vi "HEWH Reset Flow Meter.vi"(6 "Refnum in":T1, 7 "Use Emerson 5700":bool, 8 "error in (no error)":errorcluster, 9 "Debug":bool, 10 "Laurel Hot IP Address":string, 11 "dup VISA session in":refnum<visa-resource-name>) -> (0 "error out":errorcluster, 3 "VISA Refnum out":refnum<visa-resource-name>)   [LabVIEW 2016]
uses:
  Drivers/Laurel Meter/Type Definitions/Laurel Serial Commands.ctl
  Drivers/Emerson 5700 Transmitter/Type Definitions/Emerson 5700 Modbus Write Coils.ctl
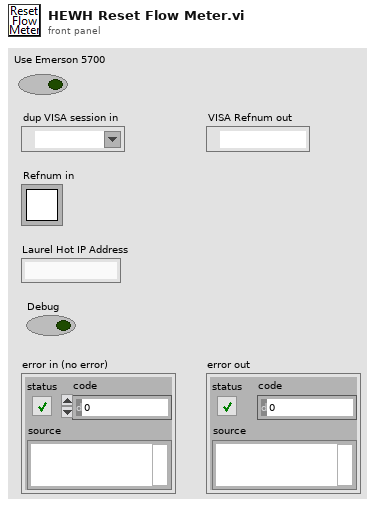
[diagram p1: front panel]
types:
  T1 = typedef "Semaphore RefNum" = refnum<k1>
  T2 = typedef "Laurel Serial Commands.ctl" = string
  T3 = enum16{"Computation Start", "Computation stop", "Reset Computation", "Clear Computation"}
  T4 = typedef "Emerson 5700 Modbus Write Coils.ctl" = u16
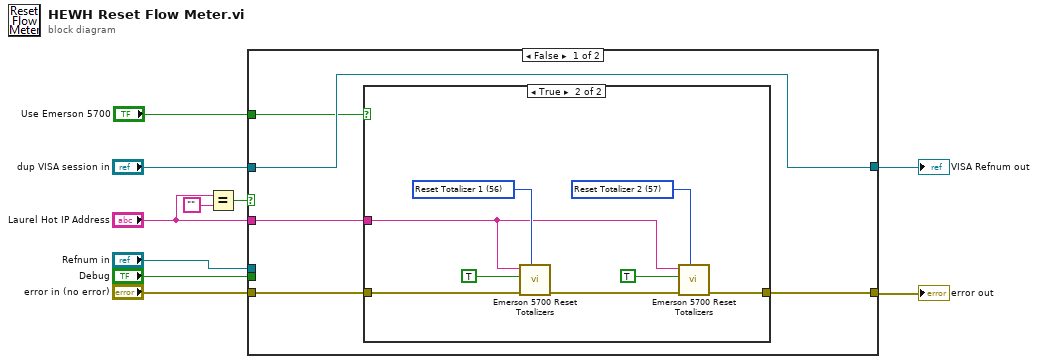
[diagram p0: block diagram]
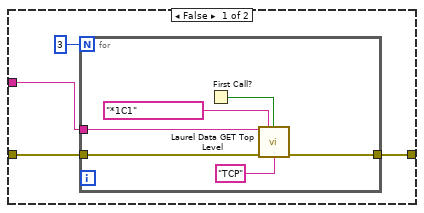
[diagram p2: hidden frame]
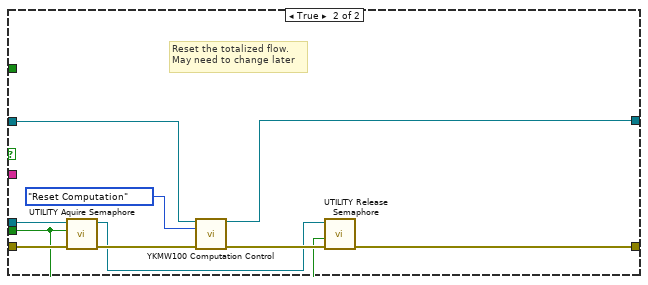
[diagram p3: hidden frame]
diagram:
  n1 = Equal?(x="Laurel Hot IP Address", y="") -> (x = y?=w3:bool)
  n2 = case shown="False" w3 {
    tunnel: "Laurel Hot IP Address" -> [w15 _]
    tunnel: "error in (no error)" -> [w14 w39]
    tunnel: [w13 w38] -> w6
    tunnel: "dup VISA session in" -> [w12 w37]
    tunnel: [w12 w36] -> w8
    tunnel: "Refnum in" -> [_ w35]
    tunnel: "Debug" -> [_ w34]
    tunnel: "Use Emerson 5700" -> [w11 _]
    frame False {
      n3 = case shown="True" w11 {
        tunnel: w15 -> [w18 w26]
        tunnel: w14 -> [w17 w33]
        tunnel: [w16 w27] -> w13
        frame False {
          n4 = for {
            N: 3 -> [_]
            tunnel: w18 -> [w20]
            tunnel: w17 -> [w22]
            tunnel: [w21] -> w16
            n5 = First Call?() -> (First Call?: T/F=w25:bool)
            n6 = call "Laurel Data GET Top Level.vi"("Laurel IP Address"=w20, "Laurel Serial Commands"=T2 "*1C1", "First Call?"=w25, "error in (no error)"=w22, "Laurel Communication Type"="TCP") -> ("error out"=w21:errorcluster)  [unwired: 5 in, 5 out]
          }
        }
        frame True {
          w29 = T4 57 items=["Start/Stop Inventory 1"=367, "Start/Stop Inventory 2"=368, "Start/Stop all Totalizers and Inventories"=2, "Reset all Totalizers"=3, "Reset all Inventories"=4, "Reset Totalizer 1"=56, "Reset Totalizer 2"=57] ("Reset all Totalizers. 2")
          w32 = T4 56 items=["Start/Stop Inventory 1"=367, "Start/Stop Inventory 2"=368, "Start/Stop all Totalizers and Inventories"=2, "Reset all Totalizers"=3, "Reset all Inventories"=4, "Reset Totalizer 1"=56, "Reset Totalizer 2"=57] ("Reset all Totalizers. 2")
          n7 = call "Emerson 5700 Reset Totalizers.vi"("Reset all Totalizers. 2"=w32, "Error In"=w33, "Coil"=TRUE, "address"=w26) -> ("Error Out"=w28:errorcluster)  [unwired: 7 in]
          n8 = call "Emerson 5700 Reset Totalizers.vi"("Reset all Totalizers. 2"=w29, "Error In"=w28, "Coil"=TRUE, "address"=w26) -> ("Error Out"=w27:errorcluster)  [unwired: 7 in]
        }
      }
    }
    frame True {
      # "Reset the totalized flow.\nMay need to change later"
      n9 = call "UTILITY Aquire Semaphore.vi"("error in (no error)"=w39, "Debug"=w34, "Refnum in"=w35) -> ("error out"=w42:errorcluster, "Refnum out"=w41:T1)  [unwired: 6 in, 1 out]
      n10 = call "YKMW100 Computation Control.vi"("VISA session"=w37, "Mode"=T3."Reset Computation", "error in (no error)"=w42) -> ("dup VISA session"=w36:refnum<visa-resource-name>, "error out"=w43:errorcluster)  [unwired: 11 in]
      n11 = call "UTILITY Release Semaphore.vi"("error in (no error)"=w43, "Debug"=w34, "Refnum in"=w41) -> ("error out"=w38:errorcluster)  [unwired: 8 in]
    }
  }
  "VISA Refnum out" <- w8
  "error out" <- w6
